vi "Write Binary Config.vi"(4 "Include Class Name":bool, 6 "byte order (0:big-endian, network order)":T1(ring), 8 "error in (no error)":errorcluster, 11 "Abs_Type in":refnum<class "Abs_Type.lvclass">) -> (0 "error out":errorcluster, 2 "Binary":string, 3 "Abs_Type out":refnum<class "Abs_Type.lvclass">)   [LabVIEW 2021, in "Abs_Type.lvclass"]
uses:
  Abs_Type.lvclass
  <vilib>/Utility/LVClass/Get LV Class Name.vi
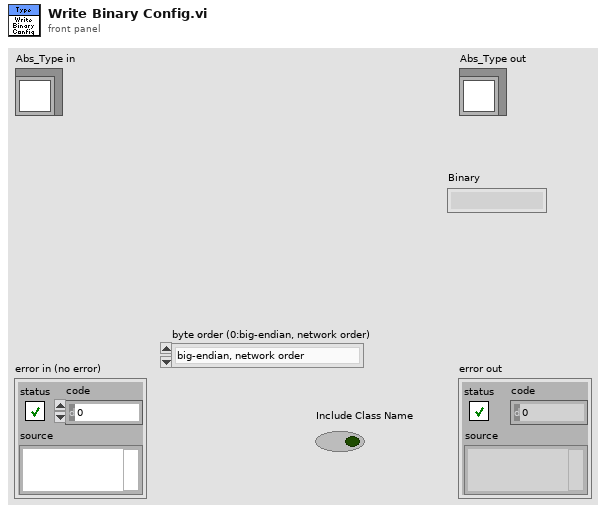
[diagram p1: front panel]
types:
  T1 = enum16{"big-endian, network order", "native, host order", "little-endian"}
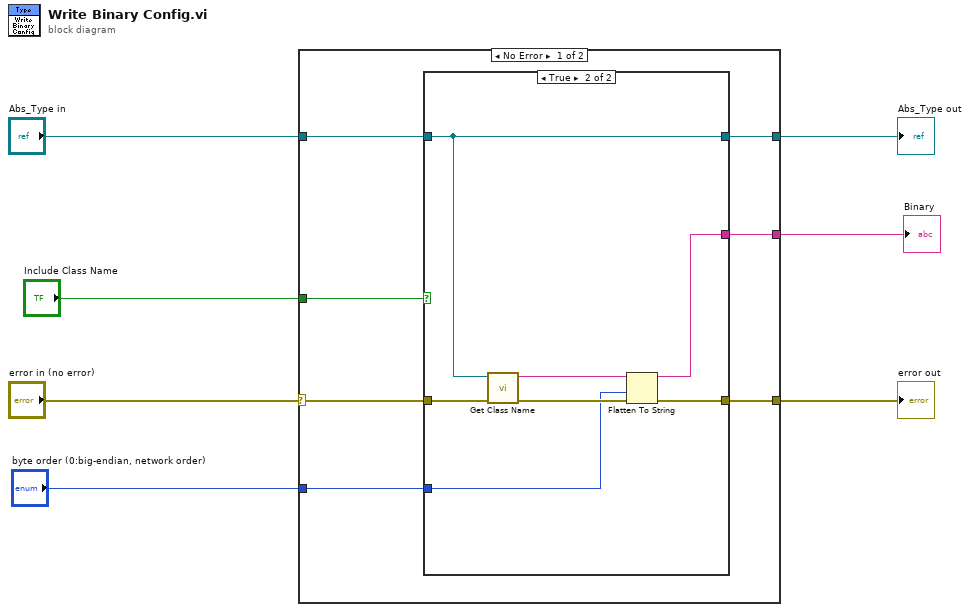
[diagram p0: block diagram]
diagram:
  n1 = case shown="No Error" "error in (no error)" {
    selector: "error in (no error)" -> [w12 w24]
    tunnel: [w9 w24] -> w6
    tunnel: "Abs_Type in" -> [w13 w25]
    tunnel: [w10 w25] -> w4
    tunnel: "Include Class Name" -> [w14 _]
    tunnel: "byte order (0:big-endian, network order)" -> [w11 _]
    tunnel: [w8 _] -> w1
    frame No Error {
      n2 = case shown="True" w14 {
        tunnel: w13 -> [w15 w19]
        tunnel: w12 -> [w16 w23]
        tunnel: w11 -> [_ w20]
        tunnel: [w15 w19] -> w10
        tunnel: [w16 w18] -> w9
        tunnel: [_ w17] -> w8
        frame False {
        }
        frame True {
          n3 = call "Get Class Name.vi"("error in (no error)"=w23, "Abs_Type in"=w19) -> ("error out"=w22:errorcluster, "class name"=w21:string)  [unwired: 8 in]
          n4 = Flatten To String(anything=w21, byte order (0:big-endian, network order)=w20, error in (no error)=w22) -> (data string=w17:string, error out=w18:errorcluster)  [unwired: 1 in, 1 out]
        }
      }
    }
    frame Error {
    }
  }
  "error out" <- w6
  "Abs_Type out" <- w4
  "Binary" <- w1
